vi "Write Setpoint.vi"(8 "error in":errorcluster, 10 "Setpoint":sgl, 11 "Alicat Device in":refnum<class "Alicat Device.lvclass">) -> (0 "error out":errorcluster, 2 "DataOut":string, 3 "Alicat Device out":refnum<class "Alicat Device.lvclass">)   [LabVIEW 2014, in "Alicat Lib.lvlib" / "Alicat Device.lvclass"]
doc: "Send a command to the controller for the setpoint. The command will be in the format <b>Xnnnnn</b> where <b>X</b> is the address and <b>nnnnn</b> is a setpoint value that ranges from 0 to 64000. The setpoint is based on the <b>Fullscale</b> value and can be calculated as\n\nnnnnn = SP*64000/FS\n\nWhen the command for a new setpoint is sent, the controller will respond with the current data values. The input <b>Setpoint</b> will be coerced in the range 0 to Full Scale."
uses:
  Alicat Device.lvclass
  Alicat Device.lvclass/Alicat Device.ctl
  Configurable Device/Configurable Device.lvclass/Configurable Device.ctl
  Configurable Device/Read Log Session.vi
  Configurable Device/Read ID.vi
  reusable/Session APIs/Serial/Public/Get Data/Get String.vi
  <userlib>/_Session Fwk/Session - Root.lvclass
  reusable/Session APIs/Serial/Serial Session.lvclass
  reusable/Session APIs/Session Log/System Log.lvclass
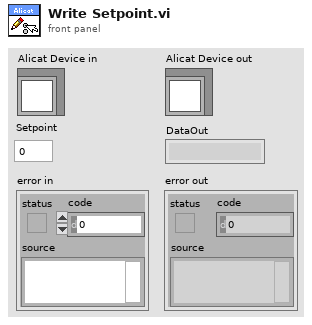
[diagram p1: front panel]
types:
  T1 = typedef "Serial Session.lvclass/Session Handle.ctl" = refnum<data-value>
  T2 = typedef "Session - Root.lvclass/Session Handle.ctl" = refnum<data-value>
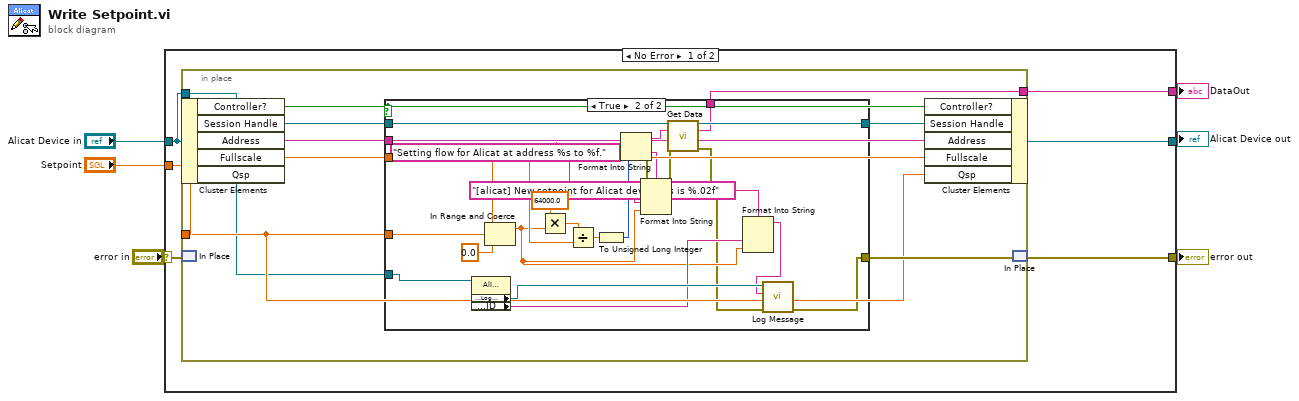
[diagram p0: block diagram]
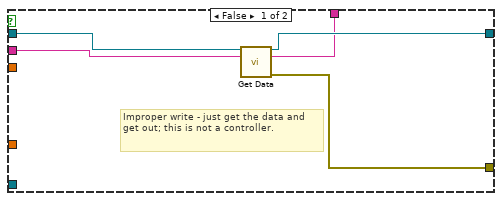
[diagram p2: hidden frame]
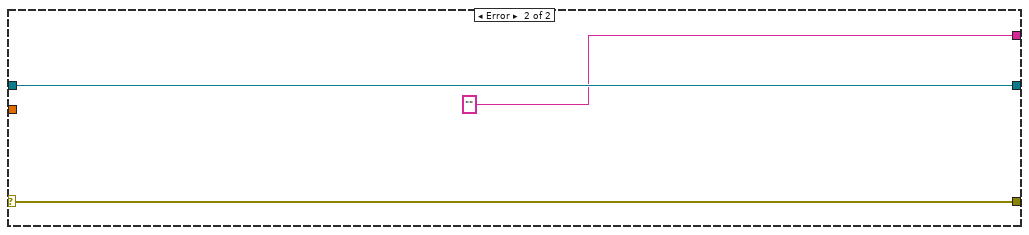
[diagram p3: hidden frame]
diagram:
  n1 = case shown="No Error" "error in" {
    selector: "error in" -> [w12 w52]
    tunnel: "Alicat Device in" -> [w7 w51]
    tunnel: [w10 w52] -> w2
    tunnel: [w11 w51] -> w3
    tunnel: [w9 "" ("DataOut")] -> w4
    tunnel: "Setpoint" -> [w8 _]
    frame No Error {
      n2 = in-place {
        in-place-border: [w18] -> w9
        in-place-border: w8 -> [w14]
        in-place-border: w7 -> [w13]
        n3 = in-place-cluster #1(w7) -> ("Controller?"=w15:bool, "Session Handle"=w21:T1, "Address"=w17:string, "Fullscale"=w16:sgl)  [unwired: 1 out]
        n4 = in-place-match #2(w12) -> ()  [unwired: 1 out]
        n5 = case shown="True" w15 {
          tunnel: w21 -> [w25 w49]
          tunnel: [w24 w48] -> w20
          tunnel: [w22 w27] -> w19
          tunnel: [w23 w47] -> w18
          tunnel: w17 -> [w26 w38]
          tunnel: w16 -> [_ w41]
          tunnel: w14 -> [_ w39]
          tunnel: w13 -> [_ w34]
          frame False {
            # "Improper write - just get the data and get out; this is not a controller."
            n6 = call-poly "Get Data.vi"("Session Handle in"=w25, "CMD"=w26) -> ("Session Handle out"=w24:T1, "DataOut"=w23:string, "error out"=w22:errorcluster)  [unwired: 11 in]
          }
          frame True {
            n7 = property class="Alicat Device"(reference=w34) -> ("Accessors:Log Session"=w33:T2, "Accessors:ID"=w31:string)  [unwired: 1 in, 2 out]
            n8 = In Range and Coerce(upper limit=w41, x=w39, lower limit=sgl 0.0) -> (coerced(x)=w30:sgl)  [unwired: 1 out]
            n9 = Multiply(x=sgl 64000.0, y=w30) -> (x*y=w45:sgl)
            n10 = Divide(x=w45, y=w41) -> (x/y=w44:sgl)
            n11 = To Unsigned Long Integer(number=w44) -> (unsigned 32bit integer=w42:u32)
            n12 = Format Into String(initial string=w38, w42) -> (resulting string=w46:string, error out=w35:errorcluster)  [unwired: 2 in]
            n13 = Format Into String(format string="Setting flow for Alicat at address %s to %f.", error in=w35, w38, w30) -> (error out=w36:errorcluster)  [unwired: 1 in, 1 out]
            n14 = call-poly "Get Data.vi"("Session Handle in"=w49, "CMD"=w46, "error in"=w36) -> ("Session Handle out"=w48:T1, "DataOut"=w47:string, "error out"=w28:errorcluster)  [unwired: 10 in]
            n15 = Format Into String(format string="[alicat] New setpoint for Alicat device %s is %.02f", w31, w30) -> (resulting string=w29:string)  [unwired: 2 in, 1 out]
            n16 = call "Log Message.vi"("error in"=w28, "MSG In"=w29, "session in"=w33) -> ("error out"=w27:errorcluster)  [unwired: 7 in, 1 out]
          }
        }
        n17 = in-place-cluster #1("Controller?"=w15, "Session Handle"=w20, "Address"=w17, "Fullscale"=w16, "Qsp"=w14) -> (w11:refnum<class "Alicat Device.lvclass">)
        n18 = in-place-match #2(w19) -> (w10:errorcluster)
      }
    }
    frame Error {
    }
  }
  "error out" <- w2
  "Alicat Device out" <- w3
  "DataOut" <- w4
